vi "CMD_CALL.vi"(8 "error in (no error)":errorcluster, 10 "Arguments":string[](array[string]), 11 "gScript Interpreter in":refnum<class "gScript Interpreter.lvclass">) -> (0 "error out":errorcluster, 3 "gScript Interpreter out":refnum<class "gScript Interpreter.lvclass">)   [LabVIEW 2017, in "gScript Interpreter.lvclass"]
uses:
  gScript Interpreter.lvclass
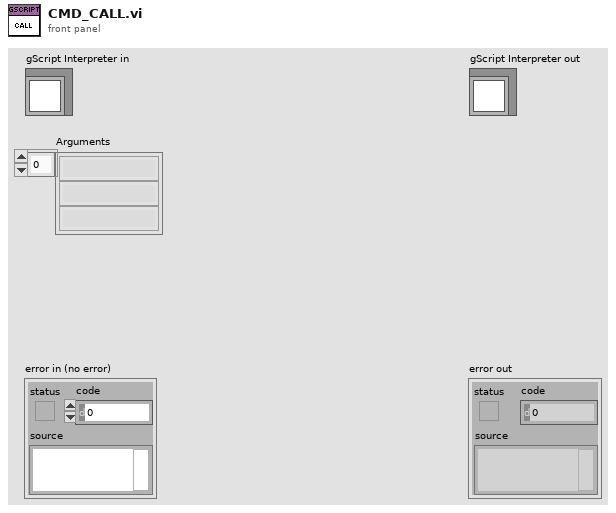
[diagram p1: front panel]
types:
  T1 = typedef "Memory Cell.ctl" = cluster{"type":T2, "x":dbl, "y":dbl, "z":dbl, "w":dbl}
  T2 = typedef "Memory Cell Type Enum.ctl" = enum16{"integer", "float", "vector", "rotation"}
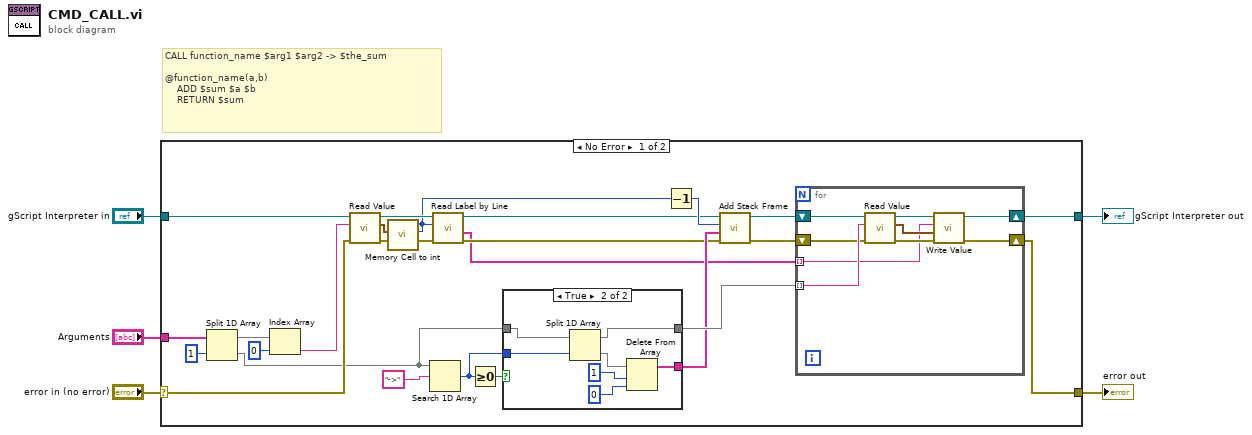
[diagram p0: block diagram]
diagram:
  # "CALL function_name $arg1 $arg2 -> $the_sum\n\n@function_name(a,b)\n    ADD $sum $a $b\n    RETURN $sum"
  n1 = case shown="No Error" "error in (no error)" {
    selector: "error in (no error)" -> [w25 w49]
    tunnel: [w21 w49] -> w4
    tunnel: [w22 w48] -> w2
    tunnel: "gScript Interpreter in" -> [w26 w48]
    tunnel: "Arguments" -> [w30 _]
    frame No Error {
      n2 = Split 1D Array(array=w30, index=1) -> (first subarray=w28:string[], second subarray=w18:string[])
      n3 = Index Array(array=w28, index=0) -> (element=w13:string)
      n4 = call-dynamic "Read Value.vi"("error in (no error)"=w25, "String in"=w13, "gScript Interpreter in"=w26) -> ("error out"=w8:errorcluster, "Memory Cell"=w11:T1, "gScript Interpreter out"=w12:refnum<class "gScript Interpreter.lvclass">)  [unwired: 6 in]
      n5 = call "Memory Cell to int.vi"("Memory Cell"=w11) -> ("Int out"=w7:i32)  [unwired: 10 in]
      n6 = Search 1D Array(1D array=w18, element="->") -> (index of element=w17:i32)  [unwired: 1 in]
      n7 = call-dynamic "Read Label by Line.vi"("error in (no error)"=w8, "Line"=w7, "gScript Interpreter in"=w12) -> ("error out"=w9:errorcluster, "Arguments"=w6:string[], "gScript Interpreter out"=w10:refnum<class "gScript Interpreter.lvclass">)  [unwired: 5 in, 1 out]
      n8 = Greater Or Equal To 0?(x=w17) -> (x >= 0?=w19:bool)
      n9 = case shown="True" w19 {
        tunnel: w18 -> [w31 w38]
        tunnel: w17 -> [_ w37]
        tunnel: [w31 w36] -> w16
        tunnel: [_ w32] -> w15
        frame False {
          # "No return bindings specified"
        }
        frame True {
          n10 = Split 1D Array(array=w38, index=w37) -> (first subarray=w36:string[], second subarray=w35:string[])
          n11 = Delete From Array(array=w35, length=1, index=0) -> (array with subset deleted=w32:string[])  [unwired: 1 out]
        }
      }
      n12 = Decrement(x=w7) -> (x-1=w14:i32)
      n13 = call "Add Stack Frame.vi"("error in (no error)"=w9, "Return Bindings"=w15, "New PC"=w14, "gScript Interpreter in"=w10) -> ("error out"=w23:errorcluster, "gScript Interpreter out"=w24:refnum<class "gScript Interpreter.lvclass">)  [unwired: 6 in]
      n14 = for {
        tunnel: w6 -> [w41] mode=indexing
        tunnel: w16 -> [w46] mode=indexing
        shift-right: [w40] -> w22
        shift-left: w24 -> [w47]
        shift-right: [w39] -> w21
        shift-left: w23 -> [w45]
        n15 = call-dynamic "Read Value.vi"("error in (no error)"=w45, "String in"=w46, "gScript Interpreter in"=w47) -> ("error out"=w43:errorcluster, "Memory Cell"=w42:T1, "gScript Interpreter out"=w44:refnum<class "gScript Interpreter.lvclass">)  [unwired: 6 in]
        n16 = call-dynamic "Write Value.vi"("error in (no error)"=w43, "Value"=w42, "Address"=w41, "gScript Interpreter in"=w44) -> ("error out"=w39:errorcluster, "gScript Interpreter out"=w40:refnum<class "gScript Interpreter.lvclass">)  [unwired: 6 in]
      }
    }
    frame Error {
    }
  }
  "error out" <- w4
  "gScript Interpreter out" <- w2
